vi "svc_Sort Peak Results.vi"(9 "sort order":u16(ring)=1 items=["Ascending", "Descending"], 10 "sort by":u16(ring)=1 items=["X", "Y"], 11 "peaks in":cluster{"X":dbl, "Y":dbl}[](array[cluster])) -> (2 "sort indices":i32[](array[numeric]), 3 "sorted peaks":cluster{"X":dbl, "Y":dbl}[](array[cluster]))   [LabVIEW 2017]
doc: "Sorts an array of peaks according to the <B>sort by</B> and <B>sort order</B> parameters. Use this VI to sort peaks that the SVFA Spectrum Peak Search, SVT Spurious Free Dynamic Range, and SVT THD and Harmonic Components VIs return. Wire data to the<B> peaks in</B> input to determine the polymorphic instance to use or manually select the instance."
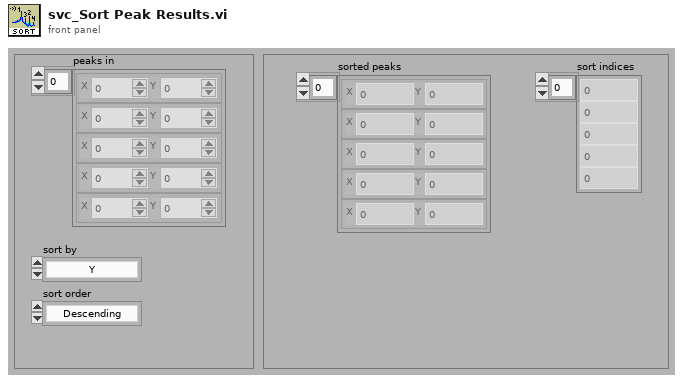
[diagram p1: front panel]
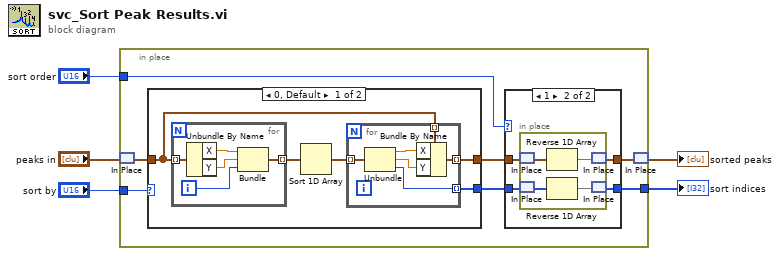
[diagram p0: block diagram]
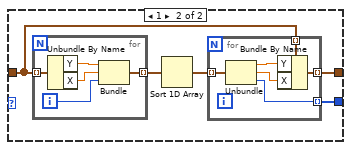
[diagram p3: hidden frame]
diagram:
  n1 = in-place {
    in-place-border: "sort by" -> [w12]
    in-place-border: "sort order" -> [w9]
    in-place-border: [w8] -> w3
    n2 = in-place-match #1("peaks in") -> (w7:cluster{"X":dbl, "Y":dbl}[])
    n3 = case shown="0, Default" w12 {
      tunnel: [w27 w42] -> w10
      tunnel: w7 -> [w23 w39]
      tunnel: [w26 w41] -> w11
      frame 0, Default {
        n4 = for {
          tunnel: [w38] -> w24 mode=indexing
          tunnel: w23 -> [w36] mode=indexing
          i -> [w37]
          n5 = Unbundle By Name(w36) -> ("X"=w35:dbl, "Y"=w34:dbl)
          n6 = Bundle("X"=w35, "Y"=w34, w37) -> (w38:cluster{"X":dbl, "Y":dbl, i32})  [unwired: 1 in]
        }
        n7 = Sort 1D Array(array=w24) -> (sorted array=w25:cluster{"X":dbl, "Y":dbl, i32}[])
        n8 = for {
          tunnel: w25 -> [w32] mode=indexing
          tunnel: [w33] -> w26 mode=indexing
          tunnel: [w29] -> w27 mode=indexing
          tunnel: w23 -> [w28] mode=indexing
          n9 = Unbundle(w32) -> ("X"=w31:dbl, "Y"=w30:dbl, w29:i32)
          n10 = Bundle By Name(cluster=w28, "X"=w31, "Y"=w30) -> (w33:cluster{"X":dbl, "Y":dbl})
        }
      }
      frame 1 {
        n11 = for {
          tunnel: [w54] -> w43 mode=indexing
          tunnel: w39 -> [w52] mode=indexing
          i -> [w53]
          n12 = Unbundle By Name(w52) -> ("Y"=w51:dbl, "X"=w50:dbl)
          n13 = Bundle("Y"=w51, "X"=w50, w53) -> (w54:cluster{"Y":dbl, "X":dbl, i32})  [unwired: 1 in]
        }
        n14 = Sort 1D Array(array=w43) -> (sorted array=w40:cluster{"Y":dbl, "X":dbl, i32}[])
        n15 = for {
          tunnel: w40 -> [w48] mode=indexing
          tunnel: [w49] -> w41 mode=indexing
          tunnel: [w45] -> w42 mode=indexing
          tunnel: w39 -> [w44] mode=indexing
          n16 = Unbundle(w48) -> ("Y"=w47:dbl, "X"=w46:dbl, w45:i32)
          n17 = Bundle By Name(cluster=w44, "Y"=w47, "X"=w46) -> (w49:cluster{"X":dbl, "Y":dbl})
        }
      }
    }
    n18 = case shown="1" w9 {
      tunnel: [w14 w17] -> w6
      tunnel: w11 -> [w14 w18]
      tunnel: w10 -> [w13 w16]
      tunnel: [w13 w15] -> w8
      frame 0, Default {
      }
      frame 1 {
        n19 = in-place {
          n20 = in-place-match #2(w18) -> (w22:cluster{"X":dbl, "Y":dbl}[])
          n21 = in-place-match #3(w16) -> (w20:i32[])
          n22 = Reverse 1D Array(array=w22) -> (reversed array=w21:cluster{"X":dbl, "Y":dbl}[])
          n23 = Reverse 1D Array(array=w20) -> (reversed array=w19:i32[])
          n24 = in-place-match #2(w21) -> (w17:cluster{"X":dbl, "Y":dbl}[])
          n25 = in-place-match #3(w19) -> (w15:i32[])
        }
      }
    }
    n26 = in-place-match #1(w6) -> (→"sorted peaks":cluster{"X":dbl, "Y":dbl}[])
  }
  "sort indices" <- w3
